vi "EnergyStorage_Read Control.vi"(11 "EnergyStorage in":refnum<class "EnergyStorage.lvclass">) -> (2 "EnergyStorage_Control":cluster{"kW setpoint":dbl}, 3 "EnergyStorage out":refnum<class "EnergyStorage.lvclass">)   [LabVIEW 2015, in "EnergyStorage.lvclass"]
uses:
  EnergyStorage.lvclass
  EnergyStorage.lvclass/EnergyStorage.ctl
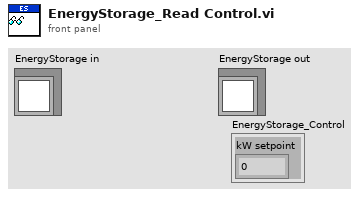
[diagram p1: front panel]
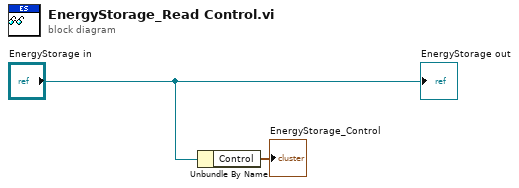
[diagram p0: block diagram]
diagram:
  n1 = Unbundle By Name("EnergyStorage in") -> ("Control"=→"EnergyStorage_Control":cluster{"kW setpoint":dbl})
  "EnergyStorage out" <- "EnergyStorage in"
